vi "Initialize Listboxes.vi"(8 "error in (no error)":errorcluster, 9 "Relay Boxes":refnum<vi>[](array[refnum]), 10 "Channel Boxes":refnum<vi>[](array[refnum]), 11 "SLSC Switch in":refnum<class "SLSC Switch.lvclass">) -> (0 "error out":errorcluster, 3 "SLSC Switch out":refnum<class "SLSC Switch.lvclass">)   [LabVIEW 2016, in "SLSC Switch.lvlib"]
uses:
  SLSC Switch.lvlib
  Classes/SLSC Switch/SLSC Switch.lvclass
  Classes/SLSC Switch/SLSC Switch.lvclass/SLSC Switch.ctl
  Classes/Switch Action Processor/Switch Action Processor.lvclass/Switch Action Processor.ctl
  Classes/Relay/Relay.lvclass/Relay.ctl
  Classes/Relay/Read name.vi
  Classes/Switch Action Processor/Read Relays.vi
  Classes/Relay/Relay.lvclass
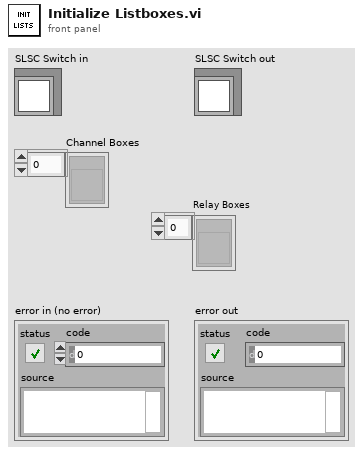
[diagram p1: front panel]
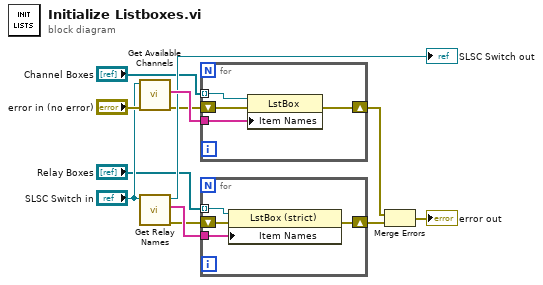
[diagram p0: block diagram]
diagram:
  n1 = call "Get Available Channels.vi"("error in (no error)"="error in (no error)", "SLSC Switch in"="SLSC Switch in") -> ("error out"=w4:errorcluster, "Channels"=w12:string[])  [unwired: 7 in, 1 out]
  n2 = call "Get Relay Names.vi"("SLSC Switch in"="SLSC Switch in") -> ("error out"=w3:errorcluster, "Relay Names"=w7:string[], "SLSC Switch out"=→"SLSC Switch out":refnum<class "SLSC Switch.lvclass">)  [unwired: 8 in]
  n3 = for {
    tunnel: w12 -> [w15]
    shift-right: [w14] -> w6
    shift-left: w4 -> [w16]
    tunnel: "Channel Boxes" -> [w13] mode=indexing
    n4 = property on="Property Node" class="LstBox"(reference=w13, error in=w16, "Item Names"=w15) -> (error out=w14:errorcluster)  [unwired: 1 out]
  }
  n5 = for {
    shift-right: [w19] -> w5
    shift-left: w3 -> [w20]
    tunnel: "Relay Boxes" -> [w18] mode=indexing
    tunnel: w7 -> [w17]
    n6 = property on="Property Node" class="LstBox (strict)"(reference=w18, error in=w20, "Item Names"=w17) -> (error out=w19:errorcluster)  [unwired: 1 out]
  }
  n7 = Merge Errors(w6, w5) -> (→"error out":errorcluster)
